vi "Pass If Equal Timestamp.vi"(6 "delta (optional)":ext, 8 "error in (no error)":errorcluster, 9 "actual timestamp":timestamp, 10 "expected timestamp":timestamp, 11 "TestCase in":refnum<class "TestCase.lvclass">) -> (0 "error out":errorcluster, 3 "TestCase out":refnum<class "TestCase.lvclass">)   [LabVIEW 2015, in "VITAC.lvlib"]
doc: "Compares two timestamps and passes if they match.\nVI internally converts timestamps to double numbers, and compares them, optionally with delta.\nIn case of failure, failure message contains exptected and actual timestamps."
uses:
  VITAC.lvlib
  <vilib>/addons/_JKI Toolkits/VI Tester/TestCase.llb/TestCase.lvclass
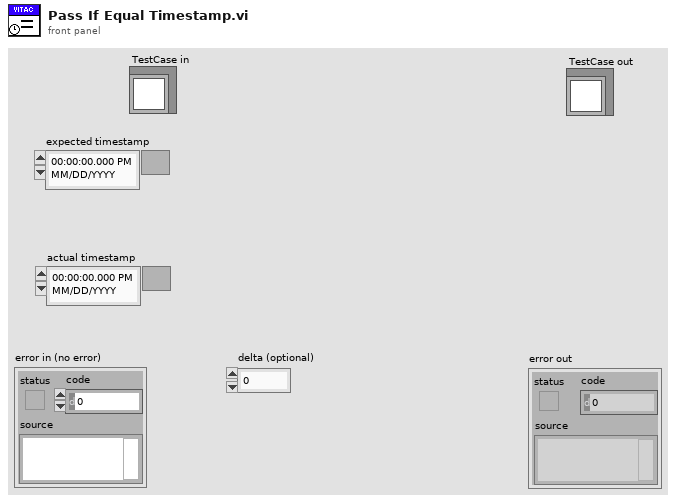
[diagram p1: front panel]
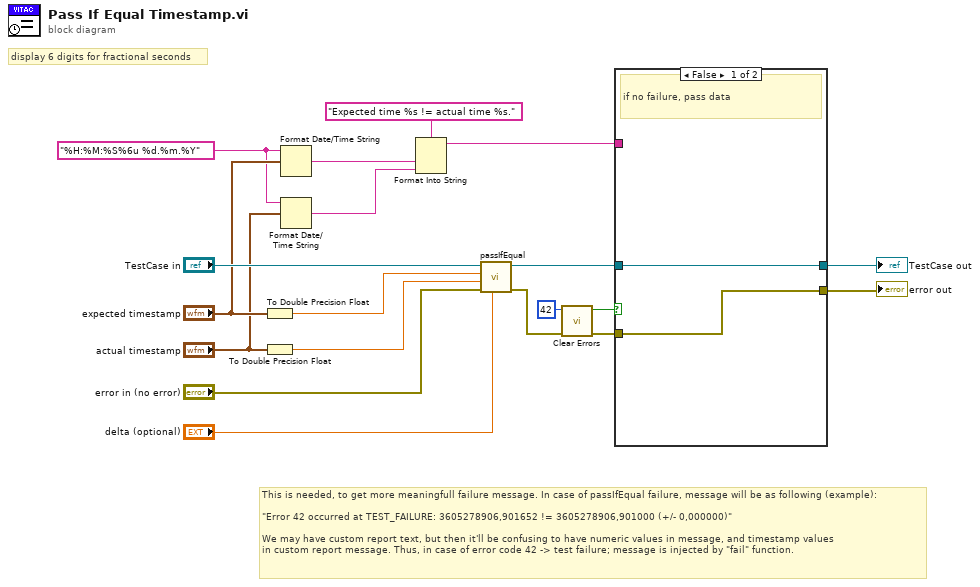
[diagram p0: block diagram]
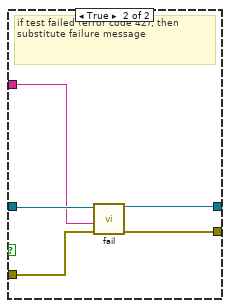
[diagram p2: hidden frame]
diagram:
  w12 = "%H:%M:%S%6u %d.%m.%Y" ("time format string (%c)")
  # "display 6 digits for fractional seconds"
  # "This is needed, to get more meaningfull failure message. In case of passIfEqual failure, message will be as following (example):\n\n\"Error 42 occurred at TEST_FAILURE: 3605278906,901652 != 3605278906,901000 (+/- 0,000000)\"\n\nWe may have custom report text, but then it'll be confusing to have numeric values in message, and timestamp values\nin custom report message. Thus, in case of error code 42 -> test failure; message is injected by \"fail\" function."
  n1 = To Double Precision Float(number="expected timestamp") -> (double precision float=w17:dbl)
  n2 = To Double Precision Float(number="actual timestamp") -> (double precision float=w16:dbl)
  n3 = Format Date/Time String(time format string (%c)=w12, seconds (now)="expected timestamp") -> (date/time string=w11:string)  [unwired: 1 in]
  n4 = Format Date/Time String(time format string (%c)=w12, seconds (now)="actual timestamp") -> (date/time string=w10:string)  [unwired: 1 in]
  n5 = Format Into String(format string="Expected time %s != actual time %s.", w11, w10) -> (resulting string=w1:string)  [unwired: 2 in, 1 out]
  n6 = call-dynamic "passIfEqual.vi"("delta (optional)"="delta (optional)", "error in (no error)"="error in (no error)", "y"=w16, "x"=w17, "TestCase in"="TestCase in") -> ("error out"=w8:errorcluster, "TestCase out"=w4:refnum<class "TestCase.lvclass">)  [unwired: 5 in]
  n7 = call <vilib>:"Clear Errors.vi"("error in (no error)"=w8, "specific error code to clear (0: all)"=42) -> ("error out"=w5:errorcluster, "specific error cleared?"=w6:bool)  [unwired: 4 in]
  n8 = case shown="False" w6 {
    tunnel: w5 -> [w20 w25]
    tunnel: w4 -> [w21 w26]
    tunnel: [w20 w24] -> w3
    tunnel: [w21 w23] -> w2
    tunnel: w1 -> [_ w22]
    frame False {
      # "if no failure, pass data"
    }
    frame True {
      # "if test failed (error code 42), then substitute failure message"
      n9 = call-dynamic "fail.vi"("error in (no error)"=w25, "message (\"\")"=w22, "TestCase in"=w26) -> ("error out"=w24:errorcluster, "TestCase out"=w23:refnum<class "TestCase.lvclass">)  [unwired: 7 in]
    }
  }
  "error out" <- w3
  "TestCase out" <- w2
